vi "niFpgaRelayTemplate.vi"(0 "input":fxp<+/-,16,16>, 1 "reset":bool, 5 "switch on point":fxp<+/-,16,16>, 7 "switch off point":fxp<+/-,16,16>, 12 "output when on":fxp<+/-,16,16>=1.0, 13 "output when off":fxp<+/-,16,16>) -> (4 "output":fxp<+/-,16,16>)   [LabVIEW 2017]
doc: "Switches between the <B>output when on</B> and <B>output when off</B> inputs. When the relay is on, it remains on until <B>input</B> is less than <B>switch off point</B>. When the relay is off, it remains off until <B>input</B> is greater than <B>switch on point</B>. The relay is off by default. The data type you wire to <B>input</B> determines the <B>output</B> data type."
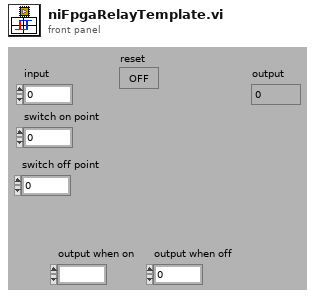
[diagram p1: front panel]
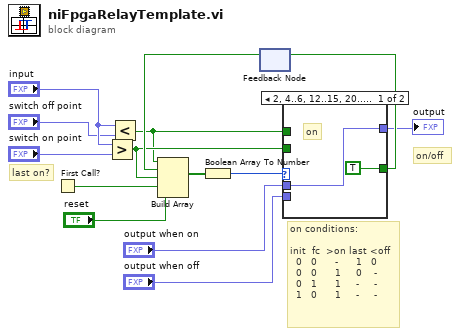
[diagram p0: block diagram]
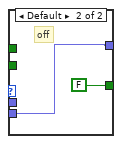
[diagram p2: hidden frame]
diagram:
  # "on conditions:\n\ninit  fc  >on last <off\n  0   0      -      1   0\n  0   0      1     0    -\n  0   1      1     -     -\n  1   0      1     -     -"
  # "on/off"
  # "last on?"
  n1 = First Call?() -> (First Call?: T/F=w13:bool)
  n2 = Greater?(x="input", y="switch on point") -> (0:w9:bool)
  n3 = Less?(x="input", y="switch off point") -> (x < y?=w7:bool)
  n4 = feedback #1() -> (w12:bool)  [unwired: 1 in]
  n5 = Build Array(w7, w12, w9, w13, "reset") -> (w11:bool[])
  n6 = Boolean Array To Number(Boolean array=w11) -> (number=w10:u8)
  n7 = case shown="2, 4..6, 12..15, 20..23" w10 {
    tunnel: [TRUE FALSE] -> w8
    tunnel: w9 -> [_ _]
    tunnel: w7 -> [_ _]
    tunnel: [w15 w17] -> w6
    tunnel: "output when on" -> [w15 _]
    tunnel: "output when off" -> [_ w17]
    frame 2, 4..6, 12..15, 20..23 {
      # "on"
    }
    frame Default {
      # "off"
    }
  }
  "output" <- w6
  n8 = feedback-in #1(w8) -> ()
